vi "UHR-Fleezers Control (fpga) - 10.3.vi"() -> ()   [LabVIEW 2009]
doc: "UHR-Fleezers Instrument Control Code (fpga)"
uses:
  <vilib>/Platform/TimedLoop/XDataNode/XDataNode.xnode
  <vilib>/Platform/TimedLoop/XDataNode/loadlvalarms.vi
  <vilib>/Platform/TimedLoop/XDataNode/timing_clust.ctl
  <vilib>/Platform/TimedLoop/XDataNode/nitl_modes.ctl
  <vilib>/Platform/TimedLoop/XDataNode/wakeup.ctl
  <vilib>/eio/EIONode/EIONode.xnode
  <vilib>/rvi/eio/nirviEIOImplementation/nirviEIOImplementation.xnode
  <vilib>/rvi/eio/common/nirviEmuTemplateMethod_noerrors.vi
  <vilib>/rvi/eio/common/nirviEmuClasses.ctl
  <vilib>/eio/EIOMethodNode/EIOMethodNode.xnode
  <vilib>/rvi/eio/nirviEIOMethodImplementation/nirviEIOMethodImplementation.xnode
  <vilib>/rvi/DataTransferAndStorage/Container/XNode/niFpgaContainer.xnode
  <vilib>/rvi/interface/RandomDataEmulation/niFpgaRandomDataHandleErrors.vi
  <vilib>/rvi/interface/RandomDataEmulation/nirviRandomDataFPGAFIFO.vi
  <vilib>/rvi/DataTransferAndStorage/Container/Common/niFpgaContainerMethod.ctl
  <vilib>/rvi/DataTransferAndStorage/Container/Common/niFpgaTransferTypeControl.ctl
  <vilib>/addons/control/pid/fpga.llb/XNode/niFpgaPID.xnode
  <vilib>/Platform/TimedLoop/XDataNode/XDNodeRunTimeDep.lvlib
panel:
  out "Trap Pos FB Int-Norm Signal":fxp<+/-,16,1> format="%.16g"
  out "Trap Pos FB Int Signal":fxp<+/-,24,9> format="%.18g"
  in  "Tab Control":T1(tab)
  in  "AI1 X Scale":u16
  in  "Trap Pos FB Monitor T1 or T2":bool
  in  "Trap Pos FB Negate Action":bool
  in  "Trap Pos. FB SP":fxp<+/-,16,1>
  in  "Trap Pos. FB Reset":bool
  in  "Trap Pos to FIFO":bool
  in  "AI1 Sets to FIFO":T2={"Set 1"=TRUE, "Set 2"=TRUE, "Set 3"=FALSE}
  in  "N of AI1 Int Acq Sets":i16=2 min=1 max=3 step=1
  out "AI Late Counter":u16
  in  "ai count":u32=400
  out "AI late?":bool
  in  "+ phase":bool
  in  "Phase count adjustment":i16
  out "Relative phase":i16
  in  "AI to FIFO":bool
  out "BD1 Frequency Out 1":u64
  out "BD1 Frequency Out 2":u64
  in  "Force feedback":bool
  out "AI1 X Set 1":fxp<+/-,16,1>
  in  "Trap Pos. FB Gains":T3={"proportional gain (Kc)"=0.0, "integral gain (Kc*Ts/Ti)"=10.0, "derivative gain (Kc*Td/Ts)"=0.0} {"proportional gain (Kc)" format="%.11g"; "integral gain (Kc*Ts/Ti)" format="%.11g"; "derivative gain (Kc*Td/Ts)" format="%.11g"}
  in  "Trap Pos. FB Range":T4={"output high"=0.999969482421875, "output low"=-1.0}
  in  "Trap Pos. FB Mult Factor":i64=2
  in  "Trap Pos. FB Offset Factor":i64
  out "AI1 X Set 2":fxp<+/-,16,1>
  out "Trap Pos FB Action":i64
  out "Trap Pos FIFO Timeout":u16
  out "Trap AI FIFO Timeout":u16
  in  "Trap FIFO Set Timeout":i32
  in  "Trap Pos FB Int Count":u16=100
  in  "Tab Control 2":T5(tab)
  in  "Swap F1 and F2":bool
  in  "Freq or Amp switch first":bool=TRUE
  in  "Cont. Scan":bool
  in  "Abort scan":bool
  in  "Cycles per step":u64
  in  "Scan BD":bool
  in  "Number of scans":u16
  in  "Scan steps":u64
  in  "Scan freq.  increment":i64
  out "Scanning":bool
  in  "Start scan":bool
  in  "OSK Bd 1":bool
  in  "Reset Bd 1":bool
  in  "RD":bool
  in  "PMODE":bool
  in  "OSK Bd 2":bool
  in  "Reset Bd 2":bool
  in  "Direct RF Box \nCommunication":bool
  in  "Data BD 2":u8 format="%08b"
  in  "Data BD 1":u8 format="%08b"
  in  "Address":u8 format="%02x"
  in  "Update Data":bool
  in  "FPGA Controls\n RF Box":bool
  in  "Number Interlace Cycles":u8=2 min=1 max=3
  in  "Interlace Off Parameters":u8=1 min=1 max=3
  in  "Interlace ON/OFF":bool
  out "DIO Relative phase":i16
  in  "Phase count adjustment (DIO)":i16
  in  "+ phase (DIO)":bool
  out "DIO Late Counter":u16
  out "DIO Late?":bool
  in  "DIO count 1 (ticks)":u32=400
  in  "DIO count 2 (ticks)":u32=400
  in  "DIO count 3 (ticks)":u32=400
  out "AI2 Y Sum Set 2":i16
  out "AI2 Y Sum Set 1":i16
  in  "FB Gains Set 1":T6={"proportional gain (Kc)"=10, "integral gain (Kc*Ts/Ti)"=5, "derivative gain (Kc*Td/Ts)"=0}
  in  "FB Setpoint Set 1":i16 min=0 step=1
  in  "FB Reset Set 1":bool
  in  "FB On/Off Set 1":bool
  in  "FB Reset Set 2":bool
  in  "FB On/Off Set 2":bool
  in  "FB Setpoint Set 2":i16 min=0 step=1
  in  "FB Gains Set 2":T6={"proportional gain (Kc)"=10, "integral gain (Kc*Ts/Ti)"=5, "derivative gain (Kc*Td/Ts)"=0}
  in  "FB output range 2":cluster{"output high":i16, "output low":i16}={"output high"=3000, "output low"=0}
  in  "FB output range 1":cluster{"output high":i16, "output low":i16}={"output high"=3000, "output low"=0}
  out "Scan I":u64
  in  "Amp switch delay":u16=5
  in  "Freq switch delay":u16
  in  "BD 2 Amplitude 1":u16
  in  "BD 1 Amplitude 1":u16
  in  "BD 2 Frequency 1":u64
  in  "BD 1 Frequency 1":u64
  in  "BD 2 Amplitude 2":u16
  in  "BD 1 Amplitude 2":u16
  in  "BD 2 Frequency 2":u64
  in  "BD 1 Frequency 2":u64
  in  "BD 2 Amplitude 3":u16
  in  "BD 1 Amplitude 3":u16
  in  "BD 2 Frequency 3":u64
  in  "BD 1 Frequency 3":u64
  out "Numeric":i32
  out "AO2 2":i16
  out "AO1 2":i16
  in  "1D or 2D Scan?":bool
  in  "Abort scan (MCL)":bool
  in  "MCL Scan Axis":bool
  in  "Cont. Scan (MCL)":bool
  out "Scan I (MCL)":u64
  in  "Number of scans (MCL)":u16
  out "Scanning MCL":bool
  in  "Scan steps (MCL)":u64
  in  "Cycles per step (MCL)":u64
  in  "Scan freq.  increment (MCL)":i16
  in  "Start scan (MCL)":bool
  in  "AO2":i16
  in  "AO1":i16
  out "MCL Late Counter":u16
  out "MCL Late?":bool
  in  "MCL count":u32=800
  out "MCL Relative Phase":i16
  in  "Phase count adjustment (MCL)":i16
  in  "+ phase (MCL)":bool
  in  "APD Gate Operating Mode":u8 max=2 step=1
  in  "Invert APD Gate":bool
  in  "APD Gate OFF Count":u32=100
  in  "APD Gate ON Count":u32=300
  out "APD 1 Gate Late Counter":u16
  out "APD 1 Gate Late?":bool
  out "APD 1 Gate Relative Phase":i16
  in  "Phase count adjustment (APD 1 Gate)":i16
  in  "+ phase (APD 1 Gate)":bool
  out "APD 2 Counts 0":u32
  out "APD 2 Counts 1":u32
  out "APD 1 Counts 0":u32
  out "APD 1 Counts 1":u32
  out "APD1 out state":bool
  in  "APD 2 AO scale factor":i16=1
  in  "APD 1 AO scale factor":i16=1
  in  "APD to FIFO":bool
  in  "APD Acq Rate Count":u32=20000000
  out "APD Acq Late Counter":u16
  out "APD Acq Late?":bool
  out "APD Acq Relative Phase":i16
  in  "Phase Count Adjustment (APD Acq)":i16
  in  "+ phase (APD Acq)":bool
  in  "Phase count adjustment (APD 2 Gate)":i16
  out "APD 2 Gate Late Counter":u16
  out "APD 2 Gate Late?":bool
  out "APD 2 Gate Relative Phase":i16
  in  "+ phase (APD 2 Gate)":bool
  out "APD2 out state":bool
  in  "Green Filter Flipper":bool
  out "Green FB Signals":T7
  in  "Green FB Count":u32=1200
  out "Green Late Counter":u16
  out "Green FB Late?":bool
  out "Green FB Relative Phase":i16
  in  "Phase count adjustment (Green FB)":i16=10
  in  "+ phase (Green FB)":bool
  out "Green FB Sum":i16
  in  "Green int current ON count adj":u32=150
  in  "Current Out":u16=30000
  in  "Green FB On/Off":bool
  in  "Green FB Setpoint":i16=250 min=0 step=1
  in  "Green FB Gains":T6={"proportional gain (Kc)"=10, "integral gain (Kc*Ts/Ti)"=5, "derivative gain (Kc*Td/Ts)"=0}
  in  "Green FB Reset":bool
  in  "Operating Mode 2":u8=2 max=2 step=1
  in  "Invert GI 2":bool
  in  "Green interlace OFF count 2":u32=900
  in  "Green interlace ON count 2":u32=300
  out "GI Late Counter 2":u16
  out "GI Late? 2":bool
  out "GI Relative phase 2":i16
  in  "Phase count adjustment (GI) 2":i16=20
  in  "+ phase (GI) 2":bool
  in  "Green interlace OFF count":u32=100
  out "GI Relative phase":i16
  in  "Phase count adjustment (GI)":i16
  in  "+ phase (GI)":bool
  out "GI Late?":bool
  in  "Green interlace ON count":u32=300
  out "GI Late Counter":u16
  in  "Invert GI":bool
  in  "Operating Mode":u8 max=2 step=1
  in  "Chassis2/Mod4/AO1":u16
  # "Only one of these can be on\nat a time:"
  # "Raster Scan AOD"
  # "1 (X)"
  # "2 (Y)"
  # "IR Intensity Feedback (RF BD 1)"
  # "AO1 (Y)"
  # "2D"
  # "1D"
  # "AO2 (X)"
  # "APD AO for aligning"
  # "Detection Loop"
  # "Green fluorescent laser digital gate interlacing loop"
  # "0 Forced ON\n1 Forced OFF\n2 Interlacing"
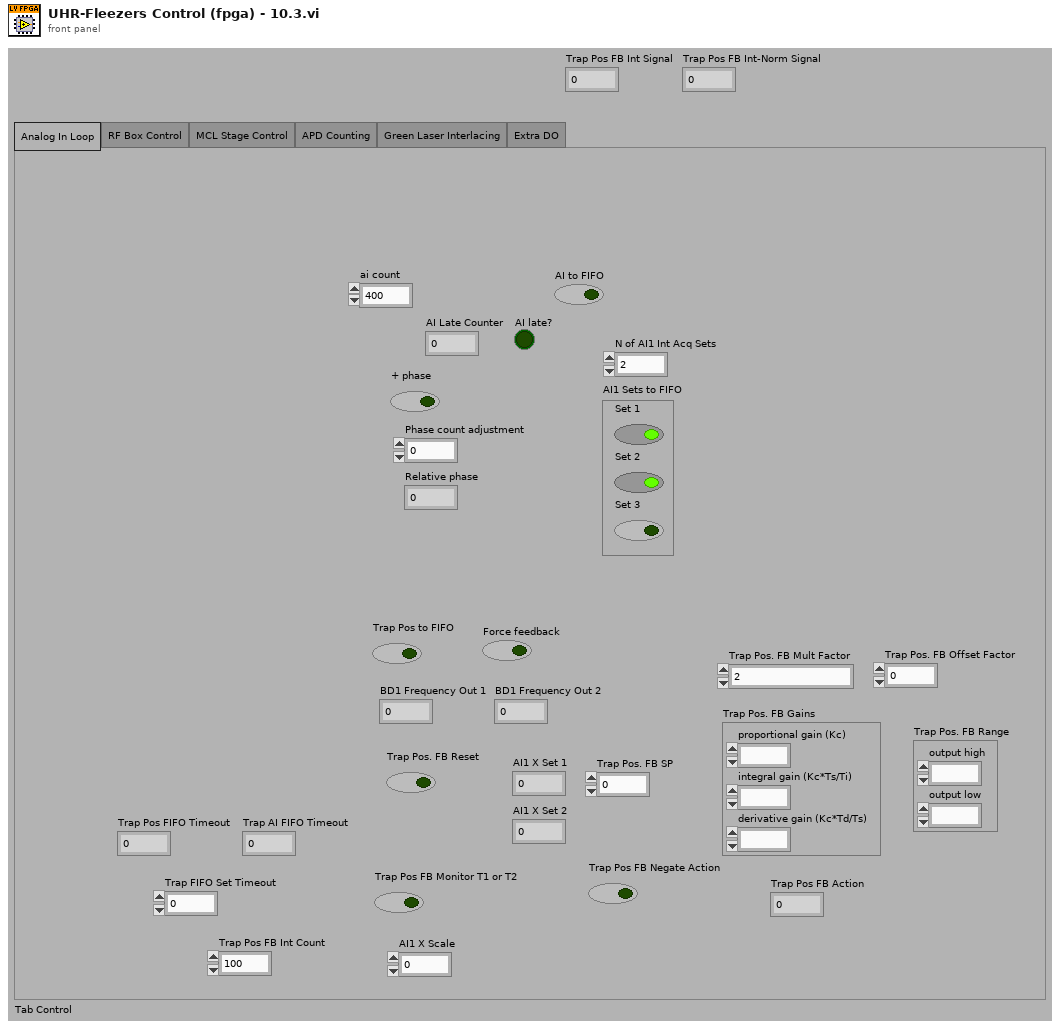
[diagram p1: front panel]
types:
  T1 = enum32{"Analog In Loop", "RF Box Control", "MCL Stage Control", "APD Counting", "Green Laser Interlacing", "Extra DO"}
  T2 = cluster{"Set 1":bool, "Set 2":bool, "Set 3":bool}
  T3 = cluster{"proportional gain (Kc)":fxp<+/-,16,8>, "integral gain (Kc*Ts/Ti)":fxp<+/-,16,8>, "derivative gain (Kc*Td/Ts)":fxp<+/-,16,8>}
  T4 = cluster{"output high":fxp<+/-,16,1>, "output low":fxp<+/-,16,1>}
  T5 = enum32{"Controls", "Interlacing Frequency and Amplitude Values"}
  T6 = cluster{"proportional gain (Kc)":i16, "integral gain (Kc*Ts/Ti)":i16, "derivative gain (Kc*Td/Ts)":i16}
  T7 = cluster{"Green FB Ch 0":i16, "Green FB Ch 1":i16, "Green FB Ch 2":i16}
  T8 = typedef "nirviEmuClasses.ctl" = enum16{"IO Read", "IO Write", "Method", "Property Read", "Property Write"}
  T9 = typedef "XDNodeRunTimeDep.lvlib/timing_clust.ctl" = cluster{"Expected End [f-1]":u64, "Actual End [f-1]":u64, "Finished Late? [f-1]":bool, "Expected End [i-1]":u64, "Actual End [i-1]":u64, "Finished Late? [i-1]":bool, "Expected Start [i]":u64, "Actual Start [i]":u64, "Expected Start [f]":u64, "Actual Start [f]":u64, "Source Name":string, "Structure Name":string, "Period":i64, "Deadline":i64, "Offset":i64, "Start":i64, "Priority":i32, "Timeout":i32, "Mode":T10, "Wakeup Reason":T11, "Error":errorcluster, "Source Type":string, "Secondary Source Type":string, "Global End Time":u64, "Global Start Time":u64, "Frame Duration":u64, "Iteration Duration":u64, "Assigned CPU":i32, "I/O Scan Engine Mode":u32}
  T10 = typedef "XDNodeRunTimeDep.lvlib/nitl_modes.ctl" = enum32{"No Change", "Process missed periods, maintain original phase", "Discard missed periods, maintain original phase", "Process missed periods, ignore original phase", "Discard missed periods, ignore original phase"}
  T11 = typedef "XDNodeRunTimeDep.lvlib/wakeup.ctl" = enum32{"Normal", "Aborted", "Asynchronous wakeup", "Timing source error", "Timed loop error", "Timeout"}
  T12 = typedef "niFpgaContainerMethod.ctl" = enum16{"Write", "Read", "Clear", "Get Number of Elements to Write", "Get Number of Elements to Read", "Enable", "Disable", "Flush and Disable", "Get Stream State"}
  T13 = typedef "niFpgaTransferTypeControl.ctl" = enum16{"Target-Scoped", "Host to Target - DMA", "Target to Host - DMA", "Peer to Peer Reader", "Peer to Peer Writer", "Bidirectional"}
  T14 = cluster{"Chassis2/Mod1/AI0":i16, "Chassis2/Mod1/AI1":i16, "Chassis2/Mod1/AI2":i16}
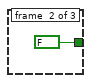
[diagram p2: hidden frame]
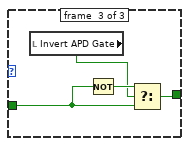
[diagram p3: hidden frame]
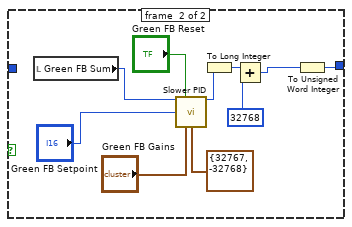
[diagram p4: hidden frame]
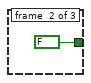
[diagram p5: hidden frame]
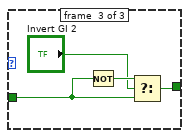
[diagram p6: hidden frame]
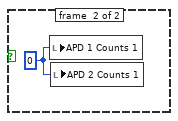
[diagram p7: hidden frame]
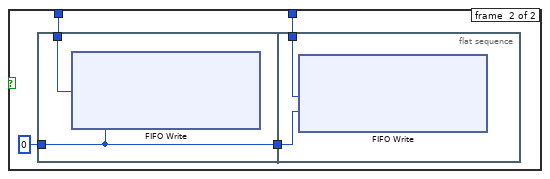
[diagram p8: hidden frame]
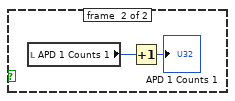
[diagram p9: hidden frame]
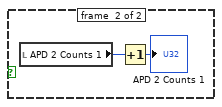
[diagram p10: hidden frame]
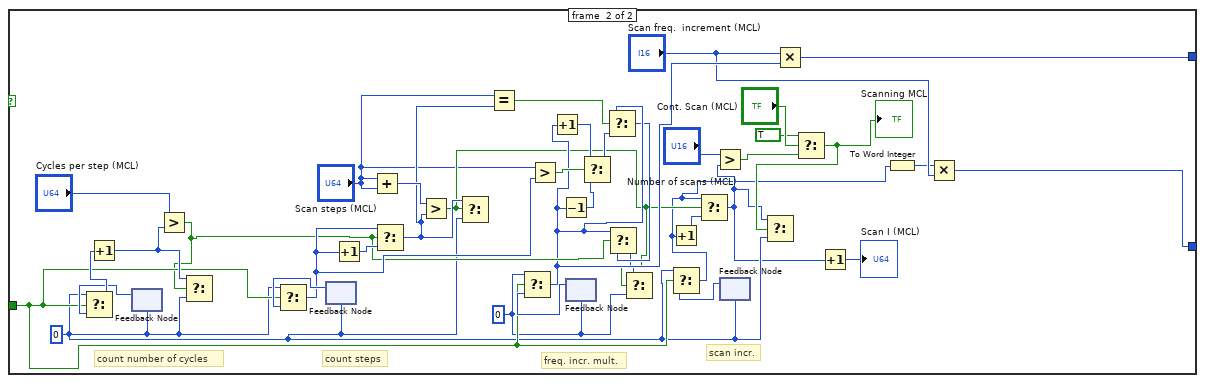
[diagram p11: hidden frame]
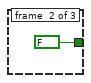
[diagram p12: hidden frame]
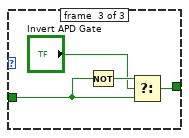
[diagram p13: hidden frame]
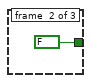
[diagram p14: hidden frame]
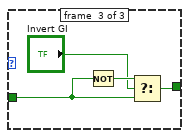
[diagram p15: hidden frame]
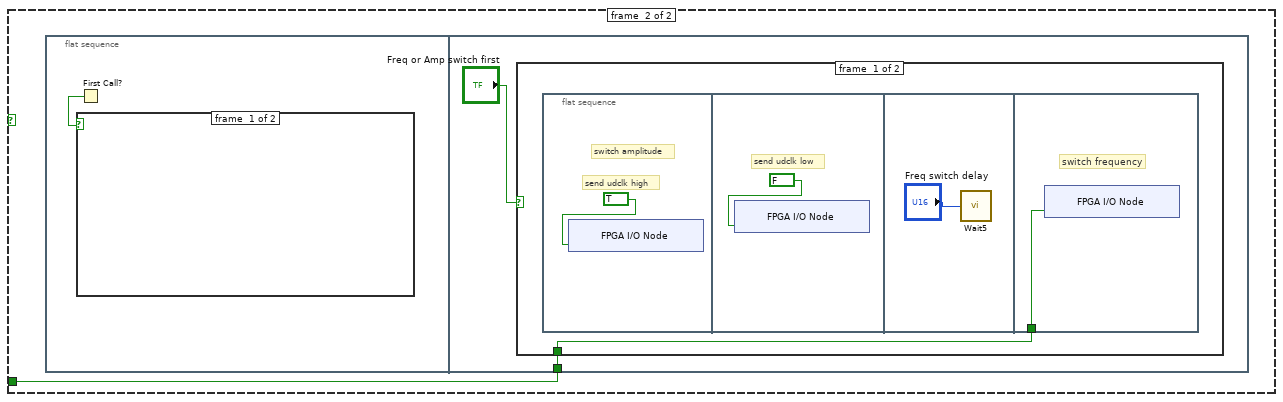
[diagram p16: hidden frame]
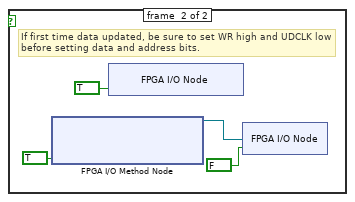
[diagram p17: hidden frame]
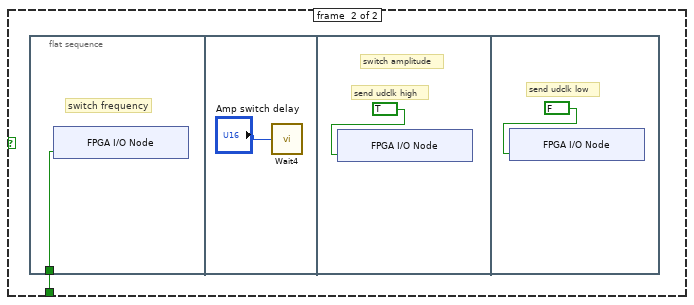
[diagram p18: hidden frame]
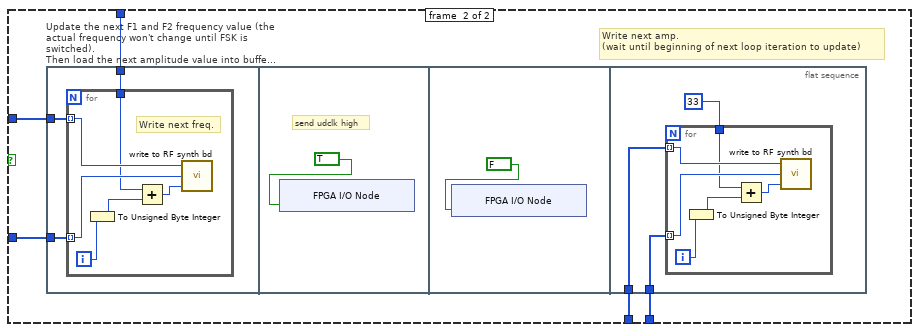
[diagram p19: hidden frame]
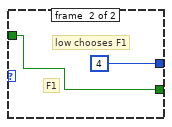
[diagram p20: hidden frame]
diagram:
  w3 = FALSE
  # "timing array current index"
  # "timing array"
  # "timing counter (phase adjusted here)"
  # "late counter"
  n1 = flat-sequence "FPGA initialization to do before running any of the loops" {
    tunnel: [u32 0 ("DIO count 3 (ticks)")] -> w2
    tunnel: [w10] -> _
    frame #0 {
      # "Start up expansion chassis early\nto avoid delays later"
      # "This pin controls udclk on the RF boards.\nWhen initially configuring the boards, this pin needs to be\nconfigured as a high impedance input.  Later it will be switched\nto an output."
      # "Initial setting of DIO data and \naddress to low (before reset).  \nThis needs to happen before the other\ncontrol method loops execute."
      n2 = xnode "FPGA I/O Node"("Chassis2/Mod4/AO0"=u16 0) -> ("Chassis2/Mod1/AI0"=w10:i16)  [unwired: 2 in, 2 out]
      n3 = xnode "FPGA I/O Method Node"("Enable"=FALSE) -> ()  [unwired: 1 in, 1 out]
      n4 = xnode "FPGA I/O Node"("Connector1/DIO0"=FALSE, "Connector1/DIO1"=FALSE, "Connector1/DIO2"=FALSE, "Connector1/DIO3"=FALSE, "Connector1/DIO4"=FALSE, "Connector1/DIO5"=FALSE, "Connector1/DIO6"=FALSE, "Connector1/DIO7"=FALSE, "Connector1/DIO8"=FALSE, "Connector1/DIO9"=FALSE, "Connector1/DIO10"=FALSE, "Connector1/DIO11"=FALSE, "Connector1/DIO12"=FALSE, "Connector1/DIO13"=FALSE, "Connector1/DIO15"=FALSE, "Connector1/DIO20"=FALSE, "Connector1/DIO21"=FALSE, "Connector1/DIO22"=FALSE, "Connector1/DIO23"=FALSE, "Connector1/DIO24"=FALSE, "Connector1/DIO25"=FALSE, "Connector1/DIO26"=FALSE, "Connector1/DIO27"=FALSE, "Connector1/DIO14"=FALSE) -> ()  [unwired: 24 in, 24 out]
    }
  }
  n5 = local read "AO1"() -> (w7:i16)
  n6 = local read "AO2"() -> (w6:i16)
  n7 = node-c288() -> (w5:T9)  [unwired: 1 in]
  n8 = while "APD 1 Counter" {
    tunnel: w2 -> [_]
    stop <- FALSE stop-if-true
    n9 = flat-sequence {
      frame #0 {
        n10 = xnode "FPGA I/O Method Node"("FPGA I/O In"=refnum<k21> "Connector0/DIO0" ("APD 1 DO"), "Timeout"=-1) -> ()  [unwired: 2 out]
      }
      frame #1 {
        n11 = local read "APD1 out state"() -> (w419:bool)
        n12 = case shown="False" w419 {
          frame #0 {
            n13 = local read "APD 1 Counts 0"() -> (w421:u32)
            n14 = Increment(x=w421) -> (x+1=→"APD 1 Counts 0":u32)
          }
          frame #1 {
            n15 = local read "APD 1 Counts 1"() -> (w423:u32)
            n16 = Increment(x=w423) -> (x+1=→"APD 1 Counts 1":u32)
          }
        }
      }
    }
  }
  n17 = while "APD 2 Counter" {
    tunnel: w2 -> [_]
    stop <- FALSE stop-if-true
    n18 = flat-sequence {
      frame #0 {
        n19 = xnode "FPGA I/O Method Node"("FPGA I/O In"=refnum<k21> "Connector0/DIO1" ("APD 2 DO"), "Timeout"=-1) -> ()  [unwired: 2 out]
      }
      frame #1 {
        n20 = local read "APD2 out state"() -> (w450:bool)
        n21 = case shown="False" w450 {
          frame #0 {
            n22 = local read "APD 2 Counts 0"() -> (w452:u32)
            n23 = Increment(x=w452) -> (x+1=→"APD 2 Counts 0":u32)
          }
          frame #1 {
            n24 = local read "APD 2 Counts 1"() -> (w454:u32)
            n25 = Increment(x=w454) -> (x+1=→"APD 2 Counts 1":u32)
          }
        }
      }
    }
  }
  n26 = while "APD 2 Gating" {
    shift-right: [w458] -> _
    shift-left: w2 -> [w463]
    shift-right: [w457] -> _
    shift-left: w3 -> [w455]
    stop <- FALSE stop-if-true
    n27 = flat-sequence {
      tunnel: w463 -> [w466]
      tunnel: [w467] -> w461
      tunnel: [w466] -> w459
      tunnel: [w465] -> w456
      tunnel: w455 -> [w465]
      tunnel: [w470] -> w462
      tunnel: w461 -> [w470]
      tunnel: [w469] -> w460
      tunnel: w459 -> [w469]
      tunnel: w456 -> [w468]
      tunnel: [w532] -> w458
      tunnel: w462 -> [w543]
      tunnel: w460 -> [w541]
      tunnel: [w536] -> w457
      frame #0 {
        n28 = call "Loop Timer8"("Count(Ticks)"=w466) -> ("Tick Count(Ticks)"=w467:u32)
      }
      frame #1 {
        # "(need 4 channels/APD)"
        n29 = xnode "FPGA I/O Node"("Connector0/DIO8"=w468, "Connector0/DIO9"=w468, "Connector0/DIO10"=w468, "Connector0/DIO11"=w468) -> ()  [unwired: 4 in, 4 out]
      }
      frame #2 {
        n30 = local read "APD Gate ON Count"() -> (w525:u32)
        n31 = local read "APD Gate OFF Count"() -> (w524:u32)
        n32 = feedback #1(TRUE) -> (w538:bool)
        n33 = feedback #2(w543) -> (w526:u32)
        n34 = Not(x=w538) -> (.not. x?=w535:bool)
        n35 = Subtract(x=w543, y=w526) -> (x-y=w542:u32)
        n36 = Select(t=w525, s=w535, f=w524) -> (s? t:f=w540:u32)
        n37 = Subtract(x=w542, y=w541) -> (x-y=w517:u32)
        n38 = Subtract(x=w540, y=w517) -> (x-y=w531:u32)
        n39 = Number To Boolean Array(number=w517) -> (Boolean array=w516:bool[])
        n40 = Or Array Elements(Boolean array=w516) -> (logical OR=w515:bool)
        "APD 2 Gate Late?" <- w515
        n41 = Boolean To (0,1)(Boolean="+ phase (APD 2 Gate)") -> (0, 1=w529:i16)
        n42 = Multiply(x=w529, y="Phase count adjustment (APD 2 Gate)") -> (x*y=w527:i16)
        n43 = Boolean To (0,1)(Boolean=w515) -> (0, 1=w522:i16)
        n44 = Add(x=w531, y=w527) -> (x+y=w532:u32)
        n45 = To Unsigned Word Integer(number=w522) -> (unsigned 16bit integer=w519:u16)
        n46 = feedback #3(i16 0) -> (w534:i16)
        n47 = Subtract(x=w534, y=w527) -> (x-y=w533:i16)
        "APD 2 Gate Relative Phase" <- w533
        n48 = feedback #4(u16 0) -> (w520:u16)
        n49 = Add(x=w519, y=w520) -> (x+y=w518:u16)
        "APD 2 Gate Late Counter" <- w518
        n50 = local read "APD Gate Operating Mode"() -> (w523:u8)
        n51 = case shown="2" w523 {
          tunnel: [TRUE FALSE w549] -> w536
          tunnel: w538 -> [_ _ w547]
          frame #0 {
          }
          frame #1 {
          }
          frame #2 {
            n52 = local read "Invert APD Gate"() -> (w546:bool)
            n53 = Not(x=w547) -> (.not. x?=w548:bool)
            n54 = Select(t=w548, s=w546, f=w547) -> (s? t:f=w549:bool)
          }
        }
      }
    }
  }
  n55 = while "DAQ AI set 1" {
    shift-right: [w550] -> _
    shift-left: w2 -> [w555]
    stop <- FALSE stop-if-true
    n56 = flat-sequence {
      tunnel: w555 -> [w565]
      tunnel: [w566] -> w553
      tunnel: [w565] -> w552
      tunnel: [w576] -> w563
      tunnel: [w575] -> w562
      tunnel: [w574] -> w561
      tunnel: [w573] -> w560
      tunnel: [w572] -> w559
      tunnel: [w571] -> w558
      tunnel: [w570] -> w557
      tunnel: [w569] -> w556
      tunnel: [w568] -> w554
      tunnel: w553 -> [w568]
      tunnel: w552 -> [w567]
      tunnel: [w567] -> w551
      tunnel: [w777] -> w550
      tunnel: w563 -> [w805]
      tunnel: w562 -> [w769]
      tunnel: w561 -> [w770]
      tunnel: w560 -> [w804]
      tunnel: w559 -> [w793]
      tunnel: w558 -> [w792]
      tunnel: w557 -> [w791]
      tunnel: w556 -> [w790]
      tunnel: w554 -> [w787]
      tunnel: w551 -> [w784]
      frame #0 {
        n57 = call "Loop Timer3"("Count(Ticks)"=w565) -> ("Tick Count(Ticks)"=w566:u32)
      }
      frame #1 {
        n58 = xnode "FPGA I/O Node"("Connector1/DIO31"=TRUE ("Connector1/DIO33")) -> ("Connector0/AI0"=w576:i16, "Connector0/AI1"=w575:i16, "Connector0/AI2"=w574:i16, "Connector0/AI3"=w573:i16, "Connector0/AI4"=w572:i16, "Connector0/AI5"=w571:i16, "Connector0/AI6"=w570:i16, "Connector0/AI7"=w569:i16)  [unwired: 9 in, 9 out]
      }
      frame #2 {
        w773 = FALSE ("AI to FIFO")
        # "Adjust phase after data acquired if button pressed"
        n59 = feedback #5(i16 1) -> (w797:i16)
        n60 = Increment(x=w797) -> (x+1=w803:i16)
        n61 = Scale By Power Of 2(n="AI1 X Scale", x=w769) -> (x*2^n=w767:i16)
        n62 = Greater?(x=w803, y="N of AI1 Int Acq Sets") -> (0:w800:bool)
        n63 = Divide(x=w767, y=w770) -> (x/y=w766:fxp<+/-,16,1>)
        n64 = Select(t=i16 1, s=w800, f=w803) -> (s? t:f=w802:i16)
        n65 = feedback #6(w773) -> (w771:bool)
        n66 = feedback #7(w773) -> (w789:bool)
        n67 = case shown="1, Default" w797 {
          tunnel: w770 -> [w852 w860 _]
          tunnel: "AI1 Sets to FIFO" -> [w856 w864 w870]
          tunnel: [w855 w863 w869] -> w794
          tunnel: ["AI to FIFO" w862 w868] -> w788
          tunnel: w789 -> [_ w862 w868]
          tunnel: ["Trap Pos to FIFO" w861 w867] -> w772
          tunnel: w771 -> [_ w861 w867]
          tunnel: w766 -> [w851 w859 _]
          tunnel: [w850 w857 FALSE] -> w753
          tunnel: [w849 w858 u64 0 ("BD1 Frequency Out 2")] -> w752
          frame #0 {
            n68 = Unbundle By Name(w856) -> ("Set 1"=w855:bool)
            n69 = local read "BD1 Frequency Out 1"() -> (w849:u64)
            n70 = Compound Arithmetic op=AND("Trap Pos to FIFO", w855, "AI to FIFO") -> (w850:bool)
            "AI2 Y Sum Set 1" <- w852
            "AI1 X Set 1" <- w851
          }
          frame #1 {
            n71 = Unbundle By Name(w864) -> ("Set 2"=w863:bool)
            n72 = local read "BD1 Frequency Out 2"() -> (w858:u64)
            n73 = Compound Arithmetic op=AND(w861, w863, w862) -> (w857:bool)
            "AI2 Y Sum Set 2" <- w860
            "AI1 X Set 2" <- w859
          }
          frame #2 {
            n74 = Unbundle By Name(w870) -> ("Set 3"=w869:bool)
          }
        }
        n75 = And(x=w794, y=w788) -> (x .and. y?=w796:bool)
        n76 = case shown="True" w796 {
          tunnel: w805 -> [_ w884]
          tunnel: w769 -> [_ w883]
          tunnel: w770 -> [_ w882]
          tunnel: w804 -> [_ w881]
          tunnel: w793 -> [_ w880]
          tunnel: w792 -> [_ w879]
          tunnel: w791 -> [_ w878]
          tunnel: w790 -> [_ w877]
          tunnel: 0 ("DMA buffer timeout") -> [_ w886]
          frame #0 {
          }
          frame #1 {
            n77 = Build Array(w884, w883, w882, w881, w880, w879, w878, w877) -> (w885:i16[])
            n78 = for {
              tunnel: w885 -> [w888] mode=indexing
              tunnel: w886 -> [w889]
              tunnel: [w887] -> w875 mode=indexing
              n79 = xnode ("FIFO Write")("Element"=w888, "Timeout"=w889) -> ("Timed Out?"=w887:bool)  [unwired: 1 in, 1 out]
            }
            n80 = Or Array Elements(Boolean array=w875) -> (logical OR=w872:bool)
            n81 = Boolean To (0,1)(Boolean=w872) -> (0, 1=w874:i16)
            n82 = feedback #8(u16 0) -> (w873:u16)
            n83 = Add(x=w874, y=w873) -> (x+y=w871:u16)
            "Trap AI FIFO Timeout" <- w871
          }
        }
        n84 = case shown="True" w753 {
          tunnel: w752 -> [_ w811]
          tunnel: [u8 0 w808] -> w751
          frame #0 {
          }
          frame #1 {
            n85 = Split Number(x=w811) -> (hi(x)=w812:u32, lo(x)=w813:u32)
            n86 = Split Number(x=w812) -> (lo(x)=w814:u16)  [unwired: 1 out]
            n87 = Split Number(x=w813) -> (hi(x)=w815:u16, lo(x)=w816:u16)
            n88 = Build Array "BD 1 nu Stack"(w814, w815, w816) -> (w810:u16[])
            n89 = for {
              tunnel: w810 -> [w823] mode=indexing
              shift-right: [w819] -> w808
              shift-left: u8 0 -> [w820]
              n90 = xnode ("FIFO Method Node")("Element"=w823, "Timeout"="Trap FIFO Set Timeout") -> ("Timed Out?"=w822:bool)  [unwired: 1 in, 1 out]
              n91 = Boolean To (0,1)(Boolean=w822) -> (0, 1=w821:i16)
              n92 = To Unsigned Byte Integer(number=w821) -> (unsigned 8bit integer=w818:u8)
              n93 = Add(x=w818, y=w820) -> (x+y=w819:u8)
            }
          }
        }
        n94 = To Unsigned Word Integer(number=w751) -> (unsigned 16bit integer=w750:u16)
        n95 = feedback #9(u16 0) -> (w764:u16)
        n96 = Add(x=w750, y=w764) -> (x+y=w763:u16)
        "Trap Pos FIFO Timeout" <- w763
        n97 = feedback #10(w787) -> (w786:u32)
        n98 = Subtract(x=w787, y=w786) -> (x-y=w785:u32)
        n99 = xnode "I/O Node"("Connector1/DIO31"=FALSE ("Connector1/DIO34")) -> ()  [unwired: 1 in, 1 out]
        n100 = Subtract(x=w785, y=w784) -> (x-y=w755:u32)
        n101 = Boolean To (0,1)(Boolean="+ phase") -> (0, 1=w780:i16)
        n102 = Multiply(x=w780, y="Phase count adjustment") -> (x*y=w774:i16)
        n103 = Subtract(x="ai count", y=w755) -> (x-y=w778:u32)
        n104 = Number To Boolean Array(number=w755) -> (Boolean array=w756:bool[])
        n105 = feedback #11(i16 0) -> (w776:i16)
        n106 = Add(x=w778, y=w774) -> (x+y=w777:u32)
        n107 = Subtract(x=w776, y=w774) -> (x-y=w775:i16)
        "Relative phase" <- w775
        n108 = Or Array Elements(Boolean array=w756) -> (logical OR=w754:bool)
        "AI late?" <- w754
        n109 = Boolean To (0,1)(Boolean=w754) -> (0, 1=w761:i16)
        n110 = To Unsigned Word Integer(number=w761) -> (unsigned 16bit integer=w758:u16)
        n111 = feedback #12(u16 0) -> (w759:u16)
        n112 = Add(x=w758, y=w759) -> (x+y=w757:u16)
        "AI Late Counter" <- w757
      }
    }
  }
  n113 = while "MCL stage control" {
    shift-right: [w943] -> _
    shift-left: w2 -> [w946]
    shift-right: [w936] -> _
    shift-left: w7 -> [w933]
    shift-right: [w935] -> _
    shift-left: w6 -> [w931]
    i -> [w930]
    stop <- FALSE stop-if-true
    n114 = flat-sequence {
      tunnel: w946 -> [w950]
      tunnel: [w951] -> w942
      tunnel: [w950] -> w940
      tunnel: [w949] -> w934
      tunnel: w933 -> [w949]
      tunnel: [w948] -> w932
      tunnel: w931 -> [w948]
      tunnel: w942 -> [w955]
      tunnel: [w955] -> w941
      tunnel: w940 -> [w954]
      tunnel: [w954] -> w939
      tunnel: w934 -> [w953]
      tunnel: w932 -> [w952]
      tunnel: [w953] -> w929
      tunnel: [w952] -> w928
      tunnel: w941 -> [w989]
      tunnel: w939 -> [w988]
      tunnel: [w989] -> w945
      tunnel: [w988] -> w944
      tunnel: [w987] -> w938
      tunnel: [w986] -> w937
      tunnel: w929 -> [w981]
      tunnel: w928 -> [w980]
      tunnel: [w1061] -> w943
      tunnel: w945 -> [w1068]
      tunnel: w944 -> [w1065]
      tunnel: w938 -> [w1063]
      tunnel: w937 -> [w1062]
      tunnel: [w1063] -> w936
      tunnel: [w1062] -> w935
      frame #0 {
        n115 = call "Loop Timer5"("Count(Ticks)"=w950) -> ("Tick Count(Ticks)"=w951:u32)
      }
      frame #1 {
        n116 = xnode "FPGA I/O Node"("Connector0/AO1"=w953, "Connector0/AO2"=w952) -> ()  [unwired: 2 in, 2 out]
      }
      frame #2 {
        n117 = local read "Scanning MCL"() -> (w1001:bool)
        n118 = Or(x=w1001, y="Start scan (MCL)") -> (x .or. y?=w996:bool)
        n119 = Not(x="Abort scan (MCL)") -> (.not. x?=w994:bool)
        n120 = And(x=w994, y=w996) -> (x .and. y?=w993:bool)
        n121 = case "Raster scan" shown="True" w993 {
          tunnel: [w1002 w1045] -> w998
          tunnel: "Start scan (MCL)" -> [_ w1030]
          tunnel: [w1002 w1006] -> w982
          frame #0 {
            w1002 = i16 0
            n122 = local write "Scanning MCL"(FALSE ("scanning")) -> ()
          }
          frame #1 {
            w1016 = i16 0
            w1015 = u64 0
            # "scan incr."
            # "freq. incr. mult."
            # "count steps"
            # "count number of cycles"
            n123 = feedback #13(w1015) -> (w1042:u64)
            n124 = Select(t=w1015, s=w1030, f=w1042) -> (s? t:f=w1044:u64)
            n125 = Increment(x=w1044) -> (x+1=w1041:u64)
            n126 = Greater?(x="Cycles per step (MCL)", y=w1041) -> (0:w1025:bool)
            n127 = Select(t=w1041, s=w1025, f=w1015) -> (s? t:f=w1040:u64)
            n128 = feedback #14(w1015) -> (w1039:u64)
            n129 = Select(t=w1015, s=w1030, f=w1039) -> (s? t:f=w1034:u64)
            n130 = Increment(x=w1034) -> (x+1=w1038:u64)
            n131 = Add(x="Scan steps (MCL)", y="Scan steps (MCL)") -> (x+y=w1037:u64)
            n132 = Select(t=w1034, s=w1025, f=w1038) -> (s? t:f=w1020:u64)
            n133 = Greater?(x=w1037, y=w1020) -> (0:w1019:bool)
            n134 = Select(t=w1020, s=w1019, f=w1015) -> (s? t:f=w1035:u64)
            n135 = Equal?(x="Scan steps (MCL)", y=w1020) -> (x = y?=w1024:bool)
            n136 = Greater?(x="Scan steps (MCL)", y=w1034) -> (0:w1033:bool)
            n137 = feedback #15(w1016) -> (w1036:i16)
            n138 = Select(t=w1016, s=w1030, f=w1036) -> (s? t:f=w1022:i16)
            n139 = Increment(x=w1022) -> (x+1=w1032:i16)
            n140 = Decrement(x=w1022) -> (x-1=w1031:i16)
            n141 = Select(t=w1032, s=w1033, f=w1031) -> (s? t:f=w1023:i16)
            n142 = Select(t=w1022, s=w1024, f=w1023) -> (s? t:f=w1021:i16)
            n143 = Select(t=w1022, s=w1025, f=w1021) -> (s? t:f=w1017:i16)
            n144 = Select(t=w1017, s=w1019, f=w1016) -> (s? t:f=w1018:i16)
            n145 = feedback #16(w1015) -> (w1029:u64)
            n146 = Select(t=w1015, s=w1030, f=w1029) -> (s? t:f=w1004:u64)
            n147 = Increment(x=w1004) -> (x+1=w1026:u64)
            n148 = Select(t=w1004, s=w1019, f=w1026) -> (s? t:f=w1005:u64)
            n149 = Greater?(x="Number of scans (MCL)", y=w1005) -> (0:w1012:bool)
            n150 = Multiply(x="Scan freq.  increment (MCL)", y=w1022) -> (x*y=w1045:i16)
            n151 = Select(t=TRUE, s="Cont. Scan (MCL)", f=w1012) -> (s? t:f=w1011:bool)
            "Scanning MCL" <- w1011
            n152 = Select(t=w1005, s=w1011, f=w1015) -> (s? t:f=w1027:u64)
            n153 = Increment(x=w1005) -> (x+1=→"Scan I (MCL)":u64)
            n154 = To Word Integer(number=w1004) -> (16bit integer=w1007:i16)
            n155 = Multiply(x=w1007, y="Scan freq.  increment (MCL)") -> (x*y=w1006:i16)
          }
        }
        n156 = Select(t=w982, s="1D or 2D Scan?", f=i16 0) -> (s? t:f=w983:i16)
        n157 = Select(t=w983, s="MCL Scan Axis", f=w998) -> (s? t:f=w997:i16)
        n158 = Select(t=w998, s="MCL Scan Axis", f=w983) -> (s? t:f=w999:i16)
        n159 = Add(x=w997, y="AO2") -> (x+y=w986:i16)
        n160 = Add(x="AO1", y=w999) -> (x+y=w987:i16)
        "AO1 2" <- w981
        "AO2 2" <- w980
      }
      frame #3 {
        n161 = feedback #17(w1068) -> (w1067:u32)
        n162 = Boolean To (0,1)(Boolean="+ phase (MCL)") -> (0, 1=w1059:i16)
        n163 = Subtract(x=w1068, y=w1067) -> (x-y=w1066:u32)
        n164 = Multiply(x=w1059, y="Phase count adjustment (MCL)") -> (x*y=w1055:i16)
        n165 = Subtract(x=w1066, y=w1065) -> (x-y=w1047:u32)
        n166 = Subtract(x="MCL count", y=w1047) -> (x-y=w1057:u32)
        n167 = feedback #18(i16 0) -> (w1056:i16)
        n168 = Subtract(x=w1056, y=w1055) -> (x-y=w1054:i16)
        "MCL Relative Phase" <- w1054
        n169 = Number To Boolean Array(number=w1047) -> (Boolean array=w1048:bool[])
        n170 = Or Array Elements(Boolean array=w1048) -> (logical OR=w1046:bool)
        "MCL Late?" <- w1046
        n171 = Boolean To (0,1)(Boolean=w1046) -> (0, 1=w1053:i16)
        n172 = Add(x=w1057, y=w1055) -> (x+y=w1061:u32)
        n173 = To Unsigned Word Integer(number=w1053) -> (unsigned 16bit integer=w1050:u16)
        n174 = feedback #19(u16 0) -> (w1051:u16)
        n175 = Add(x=w1050, y=w1051) -> (x+y=w1049:u16)
        "MCL Late Counter" <- w1049
      }
    }
    "Numeric" <- w930
  }
  n176 = while "APD 1 Gating" {
    shift-right: [w1073] -> _
    shift-left: w2 -> [w1078]
    shift-right: [w1072] -> _
    shift-left: w3 -> [w1070]
    stop <- FALSE stop-if-true
    n177 = flat-sequence {
      tunnel: w1078 -> [w1081]
      tunnel: [w1082] -> w1076
      tunnel: [w1081] -> w1074
      tunnel: [w1080] -> w1071
      tunnel: w1070 -> [w1080]
      tunnel: [w1085] -> w1077
      tunnel: w1076 -> [w1085]
      tunnel: [w1084] -> w1075
      tunnel: w1074 -> [w1084]
      tunnel: w1071 -> [w1083]
      tunnel: [w1143] -> w1073
      tunnel: w1077 -> [w1158]
      tunnel: w1075 -> [w1155]
      tunnel: [w1147] -> w1072
      frame #0 {
        n178 = call "Loop Timer7"("Count(Ticks)"=w1081) -> ("Tick Count(Ticks)"=w1082:u32)
      }
      frame #1 {
        # "(need 4 channels/APD)"
        n179 = xnode "FPGA I/O Node"("Connector0/DIO4"=w1083, "Connector0/DIO5"=w1083, "Connector0/DIO6"=w1083, "Connector0/DIO7"=w1083) -> ()  [unwired: 4 in, 4 out]
      }
      frame #2 {
        n180 = feedback #20(TRUE) -> (w1150:bool)
        n181 = feedback #21(w1158) -> (w1157:u32)
        n182 = Not(x=w1150) -> (.not. x?=w1146:bool)
        n183 = Subtract(x=w1158, y=w1157) -> (x-y=w1156:u32)
        n184 = Select(t="APD Gate ON Count", s=w1146, f="APD Gate OFF Count") -> (s? t:f=w1152:u32)
        n185 = Subtract(x=w1156, y=w1155) -> (x-y=w1131:u32)
        n186 = Subtract(x=w1152, y=w1131) -> (x-y=w1142:u32)
        n187 = Number To Boolean Array(number=w1131) -> (Boolean array=w1132:bool[])
        n188 = Or Array Elements(Boolean array=w1132) -> (logical OR=w1130:bool)
        "APD 1 Gate Late?" <- w1130
        n189 = Boolean To (0,1)(Boolean="+ phase (APD 1 Gate)") -> (0, 1=w1140:i16)
        n190 = Boolean To (0,1)(Boolean=w1130) -> (0, 1=w1137:i16)
        n191 = Multiply(x=w1140, y="Phase count adjustment (APD 1 Gate)") -> (x*y=w1138:i16)
        n192 = To Unsigned Word Integer(number=w1137) -> (unsigned 16bit integer=w1134:u16)
        n193 = Add(x=w1142, y=w1138) -> (x+y=w1143:u32)
        n194 = feedback #22(i16 0) -> (w1145:i16)
        n195 = Subtract(x=w1145, y=w1138) -> (x-y=w1144:i16)
        "APD 1 Gate Relative Phase" <- w1144
        n196 = feedback #23(u16 0) -> (w1135:u16)
        n197 = Add(x=w1134, y=w1135) -> (x+y=w1133:u16)
        "APD 1 Gate Late Counter" <- w1133
        n198 = case shown="2" "APD Gate Operating Mode" {
          tunnel: [TRUE FALSE w1164] -> w1147
          tunnel: w1150 -> [_ _ w1161]
          frame #0 {
          }
          frame #1 {
          }
          frame #2 {
            n199 = Not(x=w1161) -> (.not. x?=w1163:bool)
            n200 = Select(t=w1163, s="Invert APD Gate", f=w1161) -> (s? t:f=w1164:bool)
          }
        }
      }
    }
  }
  n201 = while "RF box board direct communication loop" {
    tunnel: w2 -> [_]
    stop <- FALSE stop-if-true
    n202 = case "Whether to use direct communication method (only use one method at a time)" shown="True" "Direct RF Box \nCommunication" {
      frame #0 {
      }
      frame #1 {
        n203 = case shown="True" "Update Data" {
          frame #0 {
          }
          frame #1 {
            n204 = flat-sequence {
              frame #0 {
                n205 = First Call?() -> (First Call?: T/F=w1168:bool)
                n206 = case shown="True" w1168 {
                  frame #0 {
                  }
                  frame #1 {
                    # "If first time data updated, be sure to set WR high\nbefore setting data and address bits."
                    n207 = flat-sequence {
                      frame #0 {
                        n208 = xnode "FPGA I/O Node"("Connector1/DIO15"=TRUE) -> ()  [unwired: 1 in, 1 out]
                      }
                      frame #1 {
                        n209 = call "Wait"("Count(Ticks)"=u8 40 ("DO Delay 3 (Ticks)")) -> ()  [unwired: 1 out]
                      }
                    }
                  }
                }
              }
              frame #1 {
                n210 = Number To Boolean Array(number="Address") -> (Boolean array=w1230:bool[])
                n211 = Number To Boolean Array(number="Data BD 1") -> (Boolean array=w1231:bool[])
                n212 = Number To Boolean Array(number="Data BD 2") -> (Boolean array=w1200:bool[])
                n213 = Index Array(array=w1231, index=7) -> (element=w1215:bool)
                n214 = Index Array(array=w1231, index=6) -> (element=w1214:bool)
                n215 = Index Array(array=w1231, index=5) -> (element=w1213:bool)
                n216 = Index Array(array=w1231, index=4) -> (element=w1212:bool)
                n217 = Index Array(array=w1231, index=3) -> (element=w1211:bool)
                n218 = Index Array(array=w1231, index=2) -> (element=w1210:bool)
                n219 = Index Array(array=w1231, index=1) -> (element=w1209:bool)
                n220 = Index Array(array=w1231, index=0) -> (element=w1208:bool)
                n221 = Index Array(array=w1230, index=5) -> (element=w1207:bool)
                n222 = Index Array(array=w1230, index=4) -> (element=w1206:bool)
                n223 = Index Array(array=w1230, index=3) -> (element=w1205:bool)
                n224 = Index Array(array=w1230, index=2) -> (element=w1204:bool)
                n225 = Index Array(array=w1230, index=1) -> (element=w1203:bool)
                n226 = Index Array(array=w1230, index=0) -> (element=w1202:bool)
                n227 = Index Array(array=w1200, index=7) -> (element=w1191:bool)
                n228 = Index Array(array=w1200, index=6) -> (element=w1190:bool)
                n229 = Index Array(array=w1200, index=5) -> (element=w1189:bool)
                n230 = Index Array(array=w1200, index=4) -> (element=w1188:bool)
                n231 = Index Array(array=w1200, index=3) -> (element=w1187:bool)
                n232 = Index Array(array=w1200, index=2) -> (element=w1186:bool)
                n233 = Index Array(array=w1200, index=1) -> (element=w1185:bool)
                n234 = Index Array(array=w1200, index=0) -> (element=w1184:bool)
                n235 = xnode "FPGA I/O Node"("Connector1/DIO0"=w1215, "Connector1/DIO1"=w1214, "Connector1/DIO2"=w1213, "Connector1/DIO3"=w1212, "Connector1/DIO4"=w1211, "Connector1/DIO5"=w1210, "Connector1/DIO6"=w1209, "Connector1/DIO7"=w1208, "Connector1/DIO8"=w1207, "Connector1/DIO9"=w1206, "Connector1/DIO10"=w1205, "Connector1/DIO11"=w1204, "Connector1/DIO12"=w1203, "Connector1/DIO13"=w1202, "Connector1/DIO20"=w1191, "Connector1/DIO21"=w1190, "Connector1/DIO22"=w1189, "Connector1/DIO23"=w1188, "Connector1/DIO24"=w1187, "Connector1/DIO25"=w1186, "Connector1/DIO26"=w1185, "Connector1/DIO27"=w1184) -> ()  [unwired: 22 in, 22 out]
              }
              frame #2 {
                # "wait and then apply write signal"
                n236 = call "Wait2"("Count(Ticks)"=u8 40 ("DO Delay 1 (Ticks)")) -> ()  [unwired: 1 out]
              }
              frame #3 {
                # "sending bit low writes data to board buffer"
                n237 = xnode "FPGA I/O Node"("Connector1/DIO15"=FALSE) -> ()  [unwired: 1 in, 1 out]
              }
              frame #4 {
                # "wait then return write signal"
                n238 = call "Wait3"("Count(Ticks)"=u8 40 ("DO Delay 2 (Ticks)")) -> ()  [unwired: 1 out]
              }
              frame #5 {
                # "sending bit high makes ready to\nwrite more data"
                n239 = xnode "FPGA I/O Node"("Connector1/DIO15"=TRUE) -> ()  [unwired: 1 in, 1 out]
              }
            }
          }
        }
      }
    }
  }
  n240 = while "Control APD data integration - stream to host" {
    shift-right: [w1552] -> _
    shift-left: w2 -> [w1557]
    stop <- FALSE stop-if-true
    n241 = flat-sequence {
      tunnel: w1557 -> [w1559]
      tunnel: [w1560] -> w1555
      tunnel: [w1559] -> w1553
      tunnel: [w1568] -> w1556
      tunnel: w1555 -> [w1568]
      tunnel: [w1567] -> w1554
      tunnel: w1553 -> [w1567]
      tunnel: [w1566] -> w1551
      tunnel: [w1565] -> w1550
      tunnel: [w1602] -> w1552
      tunnel: w1556 -> [w1614]
      tunnel: w1554 -> [w1611]
      tunnel: w1551 -> [w1595]
      tunnel: w1550 -> [w1594]
      frame #0 {
        n242 = call "Loop Timer6"("Count(Ticks)"=w1559) -> ("Tick Count(Ticks)"=w1560:u32)
      }
      frame #1 {
        n243 = flat-sequence {
          tunnel: [w1570] -> w1564
          tunnel: w1564 -> [w1572]
          tunnel: [w1574] -> w1563
          tunnel: [w1573] -> w1562
          tunnel: [w1572] -> w1561
          tunnel: [w1580] -> w1565
          tunnel: [w1581] -> w1566
          tunnel: w1563 -> [w1581]
          tunnel: w1562 -> [w1580]
          tunnel: w1561 -> [w1579]
          frame #0 {
            # "use two separate variable so each APD won't\nhave to wait to read"
            n244 = feedback #24(FALSE) -> (w1569:bool)
            "APD1 out state" <- w1569
            "APD2 out state" <- w1569
            n245 = Not(x=w1569) -> (.not. x?=w1570:bool)
          }
          frame #1 {
            n246 = local read "APD 1 Counts 1"() -> (w1578:u32)
            n247 = local read "APD 1 Counts 0"() -> (w1577:u32)
            n248 = local read "APD 2 Counts 1"() -> (w1576:u32)
            n249 = local read "APD 2 Counts 0"() -> (w1575:u32)
            n250 = Select(t=w1578, s=w1572, f=w1577) -> (s? t:f=w1574:u32)
            n251 = Select(t=w1576, s=w1572, f=w1575) -> (s? t:f=w1573:u32)
          }
          frame #2 {
            n252 = case shown="False" w1579 {
              frame #0 {
                w1582 = u32 0 ("APD 1 Counts 0")
                n253 = local write "APD 1 Counts 0"(w1582) -> ()
                n254 = local write "APD 2 Counts 0"(w1582) -> ()
              }
              frame #1 {
                w1583 = u32 0 ("APD 1 Counts 1")
                n255 = local write "APD 1 Counts 1"(w1583) -> ()
                n256 = local write "APD 2 Counts 1"(w1583) -> ()
              }
            }
          }
        }
      }
      frame #2 {
        n257 = feedback #25(w1614) -> (w1613:u32)
        n258 = Subtract(x=w1614, y=w1613) -> (x-y=w1612:u32)
        n259 = Subtract(x=w1612, y=w1611) -> (x-y=w1587:u32)
        n260 = case shown="True" "APD to FIFO" {
          tunnel: w1595 -> [_ w1641]
          tunnel: w1594 -> [_ w1639]
          frame #0 {
          }
          frame #1 {
            n261 = flat-sequence {
              tunnel: 0 ("Timeout") -> [w1643]
              tunnel: w1641 -> [w1644]
              tunnel: [w1643] -> w1640
              tunnel: w1640 -> [w1671]
              tunnel: w1639 -> [w1670]
              frame #0 {
                n262 = xnode ("FIFO Write")("Element"=w1644, "Timeout"=w1643) -> ()  [unwired: 1 in, 2 out]
              }
              frame #1 {
                n263 = xnode ("FIFO Write")("Element"=w1670, "Timeout"=w1671) -> ()  [unwired: 1 in, 2 out]
              }
            }
          }
        }
        n264 = Subtract(x="APD Acq Rate Count", y=w1587) -> (x-y=w1603:u32)
        n265 = Number To Boolean Array(number=w1587) -> (Boolean array=w1588:bool[])
        n266 = Or Array Elements(Boolean array=w1588) -> (logical OR=w1586:bool)
        "APD Acq Late?" <- w1586
        n267 = Boolean To (0,1)(Boolean=w1586) -> (0, 1=w1593:i16)
        n268 = To Unsigned Word Integer(number=w1593) -> (unsigned 16bit integer=w1590:u16)
        n269 = Boolean To (0,1)(Boolean="+ phase (APD Acq)") -> (0, 1=w1599:i16)
        n270 = feedback #26(u16 0) -> (w1591:u16)
        n271 = Add(x=w1590, y=w1591) -> (x+y=w1589:u16)
        "APD Acq Late Counter" <- w1589
        n272 = Multiply(x=w1599, y="Phase Count Adjustment (APD Acq)") -> (x*y=w1596:i16)
        n273 = Add(x=w1603, y=w1596) -> (x+y=w1602:u32)
        n274 = feedback #27(i16 0) -> (w1601:i16)
        n275 = Subtract(x=w1601, y=w1596) -> (x-y=w1598:i16)
        "APD Acq Relative Phase" <- w1598
        n276 = To Word Integer(number=w1595) -> (16bit integer=w1604:i16)
        n277 = To Word Integer(number=w1594) -> (16bit integer=w1605:i16)
        n278 = Multiply(x="APD 1 AO scale factor", y=w1604) -> (x*y=w1585:i16)
        n279 = Multiply(x="APD 2 AO scale factor", y=w1605) -> (x*y=w1584:i16)
        n280 = xnode "FPGA I/O Node"("Connector0/AO6"=w1585, "Connector0/AO7"=w1584) -> ()  [unwired: 2 in, 2 out]
      }
    }
  }
  n281 = timed-loop "RF box board DIO control: control bits" {
    timing: w5 -> [_]
    timing-out: [_] -> w4
    tunnel: [w1697] -> _
    tunnel: w2 -> [w1697]
    stop <- FALSE stop-if-true
    n282 = xnode "FPGA I/O Node"("Connector1/DIO16"="RD", "Connector1/DIO17"="PMODE", "Connector1/DIO18"="OSK Bd 1", "Connector1/DIO19"="Reset Bd 1", "Connector1/DIO28"="OSK Bd 2", "Connector1/DIO29"="Reset Bd 2") -> ()  [unwired: 6 in, 6 out]
  }
  n283 = while "Green fluorescent laser interlacing (DO to IA 532 nm AOM ME amp)." {
    shift-right: [w1788] -> _
    shift-left: w2 -> [w1793]
    shift-right: [w1787] -> _
    shift-left: FALSE -> [w1785]
    stop <- FALSE stop-if-true
    n284 = flat-sequence {
      tunnel: w1793 -> [w1796]
      tunnel: [w1797] -> w1791
      tunnel: [w1796] -> w1789
      tunnel: [w1795] -> w1786
      tunnel: w1785 -> [w1795]
      tunnel: [w1800] -> w1792
      tunnel: w1791 -> [w1800]
      tunnel: [w1799] -> w1790
      tunnel: w1789 -> [w1799]
      tunnel: w1786 -> [w1798]
      tunnel: [w1848] -> w1788
      tunnel: w1792 -> [w1868]
      tunnel: w1790 -> [w1865]
      tunnel: [w1857] -> w1787
      frame #0 {
        n285 = call "Loop Timer4"("Count(Ticks)"=w1796) -> ("Tick Count(Ticks)"=w1797:u32)
      }
      frame #1 {
        n286 = xnode "FPGA I/O Node"("Connector1/DIO37"=w1798, "Connector1/DIO38"=w1798, "Connector1/DIO39"=w1798) -> ()  [unwired: 3 in, 3 out]
      }
      frame #2 {
        n287 = feedback #28(w1868) -> (w1867:u32)
        n288 = Subtract(x=w1868, y=w1867) -> (x-y=w1866:u32)
        n289 = Subtract(x=w1866, y=w1865) -> (x-y=w1841:u32)
        n290 = Number To Boolean Array(number=w1841) -> (Boolean array=w1842:bool[])
        n291 = Or Array Elements(Boolean array=w1842) -> (logical OR=w1840:bool)
        "GI Late?" <- w1840
        n292 = Boolean To (0,1)(Boolean="+ phase (GI)") -> (0, 1=w1853:i16)
        n293 = Multiply(x=w1853, y="Phase count adjustment (GI)") -> (x*y=w1850:i16)
        n294 = Boolean To (0,1)(Boolean=w1840) -> (0, 1=w1847:i16)
        n295 = To Unsigned Word Integer(number=w1847) -> (unsigned 16bit integer=w1844:u16)
        n296 = feedback #29(i16 0) -> (w1851:i16)
        n297 = feedback #30(u16 0) -> (w1845:u16)
        n298 = Add(x=w1844, y=w1845) -> (x+y=w1843:u16)
        "GI Late Counter" <- w1843
        n299 = Subtract(x=w1851, y=w1850) -> (x-y=w1849:i16)
        "GI Relative phase" <- w1849
        n300 = feedback #31(TRUE) -> (w1860:bool)
        n301 = case shown="2" "Operating Mode" {
          tunnel: [TRUE FALSE w1874] -> w1857
          tunnel: w1860 -> [_ _ w1871]
          frame #0 {
          }
          frame #1 {
          }
          frame #2 {
            n302 = Not(x=w1871) -> (.not. x?=w1873:bool)
            n303 = Select(t=w1873, s="Invert GI", f=w1871) -> (s? t:f=w1874:bool)
          }
        }
        n304 = Not(x=w1860) -> (.not. x?=w1856:bool)
        n305 = Select(t="Green interlace ON count", s=w1856, f="Green interlace OFF count") -> (s? t:f=w1862:u32)
        n306 = Subtract(x=w1862, y=w1841) -> (x-y=w1854:u32)
        n307 = Add(x=w1854, y=w1850) -> (x+y=w1848:u32)
      }
    }
  }
  n308 = while "Green fluorescent laser interlacing (Current to IA 532 nm AOM ME amp)." {
    shift-right: [w1880] -> _
    shift-left: w2 -> [w1883]
    shift-right: [w1877] -> _
    shift-left: u16 0 -> [w1875]
    stop <- FALSE stop-if-true
    n309 = flat-sequence {
      tunnel: w1883 -> [w1886]
      tunnel: [w1887] -> w1882
      tunnel: [w1886] -> w1881
      tunnel: [w1885] -> w1876
      tunnel: w1875 -> [w1885]
      tunnel: [w1890] -> w1879
      tunnel: w1882 -> [w1890]
      tunnel: [w1889] -> w1878
      tunnel: w1881 -> [w1889]
      tunnel: w1876 -> [w1888]
      tunnel: [w1911] -> w1880
      tunnel: [w1928] -> w1877
      tunnel: w1879 -> [w1941]
      tunnel: w1878 -> [w1938]
      frame #0 {
        n310 = call "Loop Timer10"("Count(Ticks)"=w1886) -> ("Tick Count(Ticks)"=w1887:u32)
      }
      frame #1 {
        n311 = xnode "FPGA I/O Node"("Chassis2/Mod4/AO0"=w1888) -> ()  [unwired: 1 in, 1 out]
      }
      frame #2 {
        n312 = Subtract(x="Green interlace OFF count 2", y="Green int current ON count adj") -> (x-y=w1920:u32)
        n313 = feedback #32(w1941) -> (w1940:u32)
        n314 = Add(x="Green int current ON count adj", y="Green interlace ON count 2") -> (x+y=w1921:u32)
        n315 = Subtract(x=w1941, y=w1940) -> (x-y=w1939:u32)
        n316 = Subtract(x=w1939, y=w1938) -> (x-y=w1904:u32)
        n317 = Number To Boolean Array(number=w1904) -> (Boolean array=w1905:bool[])
        n318 = Boolean To (0,1)(Boolean="+ phase (GI) 2") -> (0, 1=w1917:i16)
        n319 = Or Array Elements(Boolean array=w1905) -> (logical OR=w1903:bool)
        "GI Late? 2" <- w1903
        n320 = Boolean To (0,1)(Boolean=w1903) -> (0, 1=w1910:i16)
        n321 = Multiply(x=w1917, y="Phase count adjustment (GI) 2") -> (x*y=w1913:i16)
        n322 = To Unsigned Word Integer(number=w1910) -> (unsigned 16bit integer=w1906:u16)
        n323 = feedback #33(u16 0) -> (w1908:u16)
        n324 = Add(x=w1906, y=w1908) -> (x+y=w1907:u16)
        "GI Late Counter 2" <- w1907
        n325 = feedback #34(i16 0) -> (w1914:i16)
        n326 = Subtract(x=w1914, y=w1913) -> (x-y=w1912:i16)
        "GI Relative phase 2" <- w1912
        n327 = feedback #35(TRUE) -> (w1933:bool)
        n328 = case shown="2" "Operating Mode 2" {
          tunnel: [TRUE FALSE w1958] -> w1922
          tunnel: w1933 -> [_ _ w1955]
          frame #0 {
          }
          frame #1 {
          }
          frame #2 {
            n329 = Not(x=w1955) -> (.not. x?=w1957:bool)
            n330 = Select(t=w1957, s="Invert GI 2", f=w1955) -> (s? t:f=w1958:bool)
          }
        }
        n331 = And(x=w1922, y="Green FB On/Off") -> (x .and. y?=w1923:bool)
        n332 = case shown="True" w1923 {
          tunnel: "Current Out" -> [w1942 _]
          tunnel: [w1942 w1947] -> w1927
          frame #0 {
          }
          frame #1 {
            n333 = local read "Green FB Sum"() -> (w1943:i16)
            n334 = call "Slower PID.vi"("process variable"=w1943, "reset?"="Green FB Reset", "setpoint"="Green FB Setpoint", "PID gains (x 2^8)"="Green FB Gains", "output range"=cluster{"output high":i16, "output low":i16} {"output high"=32767, "output low"=-32768} ("Green FB output range")) -> ("output"=w1951:i16)  [unwired: 10 out]
            n335 = To Long Integer(number=w1951) -> (32bit integer=w1944:i32)
            n336 = Add(x=w1944, y=32768) -> (x+y=w1946:i32)
            n337 = To Unsigned Word Integer(number=w1946) -> (unsigned 16bit integer=w1947:u16)
          }
        }
        n338 = Not(x=w1933) -> (.not. x?=w1930:bool)
        n339 = Select(t=w1921, s=w1930, f=w1920) -> (s? t:f=w1935:u32)
        n340 = Subtract(x=w1935, y=w1904) -> (x-y=w1915:u32)
        n341 = Add(x=w1915, y=w1913) -> (x+y=w1911:u32)
        n342 = Boolean To (0,1)(Boolean=w1922) -> (0, 1=w1929:i16)
        n343 = To Unsigned Word Integer(number=w1929) -> (unsigned 16bit integer=w1926:u16)
        n344 = Multiply(x=w1926, y=w1927) -> (x*y=w1928:u16)
      }
    }
  }
  n345 = while "Green excitation laser feedback measurement" {
    shift-right: [w1959] -> _
    shift-left: w2 -> [w1964]
    stop <- FALSE stop-if-true
    n346 = flat-sequence {
      tunnel: w1964 -> [w1966]
      tunnel: [w1967] -> w1962
      tunnel: [w1966] -> w1960
      tunnel: [w1974] -> w1963
      tunnel: w1962 -> [w1974]
      tunnel: [w1973] -> w1961
      tunnel: w1960 -> [w1973]
      tunnel: [w2058] -> w1959
      tunnel: w1963 -> [w2069]
      tunnel: w1961 -> [w2066]
      frame #0 {
        n347 = call "Loop Timer9"("Count(Ticks)"=w1966) -> ("Tick Count(Ticks)"=w1967:u32)
      }
      frame #1 {
        n348 = xnode "FPGA I/O Node"("Connector1/DIO35"=TRUE) -> ("Chassis2/Mod1/AI0"=w1972:i16, "Chassis2/Mod1/AI1"=w1971:i16, "Chassis2/Mod1/AI2"=w1968:i16)  [unwired: 4 in, 4 out]
        "Green FB Sum" <- w1968
        n349 = Bundle("Chassis2/Mod1/AI0"=w1972, "Chassis2/Mod1/AI1"=w1971, "Chassis2/Mod1/AI2"=w1968) -> (→"Green FB Signals":T14)  [unwired: 1 out]
      }
      frame #2 {
        n350 = feedback #36(w2069) -> (w2068:u32)
        n351 = Subtract(x=w2069, y=w2068) -> (x-y=w2067:u32)
        n352 = xnode "FPGA I/O Node"("Connector1/DIO35"=FALSE) -> ()  [unwired: 1 in, 1 out]
        n353 = Subtract(x=w2067, y=w2066) -> (x-y=w2048:u32)
        n354 = Subtract(x="Green FB Count", y=w2048) -> (x-y=w2062:u32)
        n355 = Number To Boolean Array(number=w2048) -> (Boolean array=w2049:bool[])
        n356 = Or Array Elements(Boolean array=w2049) -> (logical OR=w2047:bool)
        "Green FB Late?" <- w2047
        n357 = Boolean To (0,1)(Boolean="+ phase (Green FB)") -> (0, 1=w2060:i16)
        n358 = Boolean To (0,1)(Boolean=w2047) -> (0, 1=w2054:i16)
        n359 = Multiply(x=w2060, y="Phase count adjustment (Green FB)") -> (x*y=w2055:i16)
        n360 = Add(x=w2062, y=w2055) -> (x+y=w2058:u32)
        n361 = To Unsigned Word Integer(number=w2054) -> (unsigned 16bit integer=w2051:u16)
        n362 = feedback #37(i16 0) -> (w2057:i16)
        n363 = Subtract(x=w2057, y=w2055) -> (x-y=w2056:i16)
        "Green FB Relative Phase" <- w2056
        n364 = feedback #38(u16 0) -> (w2052:u16)
        n365 = Add(x=w2051, y=w2052) -> (x+y=w2050:u16)
        "Green Late Counter" <- w2050
      }
    }
  }
  n366 = while "Control Additional IO (Green laser flip mount)" {
    stop <- FALSE stop-if-true
    n367 = xnode "FPGA I/O Node"("Connector0/DIO3"="Green Filter Flipper", "Chassis2/Mod4/AO1"="Chassis2/Mod4/AO1") -> ()  [unwired: 2 in, 2 out]
    n368 = call "Loop Timer2"("Count(Ticks)"=u32 40000 ("Extra DO Counts")) -> ()  [unwired: 1 out]
  }
  n369 = while "RF box board DIO control: parallel communication" {
    shift-right: [w2114] -> _
    shift-left: w2 -> [w2113]
    shift-right: [w2112] -> _
    shift-left: FALSE ("Swap F1 and F2") -> [w2111]
    stop <- FALSE stop-if-true
    n370 = flat-sequence {
      tunnel: w2111 -> [w2118]
      tunnel: w2113 -> [w2116]
      tunnel: [w2118] -> w2110
      tunnel: [w2117] -> w2109
      tunnel: [w2116] -> w2108
      tunnel: [w2124] -> w2114
      tunnel: [w2123] -> w2112
      tunnel: w2110 -> [w2122]
      tunnel: w2109 -> [w2120]
      tunnel: w2108 -> [w2119]
      frame #0 {
        n371 = call "Loop Timer"("Count(Ticks)"=w2116) -> ("Tick Count(Ticks)"=w2117:u32)
      }
      frame #1 {
        n372 = flat-sequence {
          tunnel: ["FPGA Controls\n RF Box"] -> w2121
          tunnel: w2122 -> [w2125]
          tunnel: [w2282] -> w2124
          tunnel: [w2295] -> w2123
          tunnel: w2121 -> [w2294]
          tunnel: w2120 -> [w2288]
          tunnel: w2119 -> [w2285]
          frame #0 {
            n373 = case shown="True" "FPGA Controls\n RF Box" {
              tunnel: w2125 -> [_ w2127]
              frame #0 {
              }
              frame #1 {
                n374 = flat-sequence {
                  tunnel: w2127 -> [w2172]
                  frame #0 {
                    n375 = First Call?() -> (First Call?: T/F=w2128:bool)
                    n376 = case shown="True" w2128 {
                      frame #0 {
                      }
                      frame #1 {
                        # "If first time data updated, be sure to set WR high and UDCLK low\nbefore setting data and address bits."
                        n377 = xnode "FPGA I/O Method Node"("Enable"=TRUE) -> ("FPGA I/O Out"=w2130:refnum<k21>)  [unwired: 1 in]
                        n378 = xnode "FPGA I/O Node"("Connector1/DIO15"=TRUE) -> ()  [unwired: 1 in, 1 out]
                        n379 = xnode "FPGA I/O Node"("I/O Item"=FALSE ("Connector1/DIO30"), "FPGA I/O In"=w2130) -> ()  [unwired: 1 out]
                      }
                    }
                  }
                  frame #1 {
                    n380 = case shown="True" "Freq or Amp switch first" {
                      tunnel: w2172 -> [w2174 w2218]
                      frame #0 {
                        n381 = flat-sequence {
                          tunnel: w2174 -> [w2204]
                          frame #0 {
                            # "switch amplitude"
                            # "send udclk high"
                            n382 = xnode "FPGA I/O Node"("Connector1/DIO30"=TRUE ("Connector1/DIO15")) -> ()  [unwired: 1 in, 1 out]
                          }
                          frame #1 {
                            # "send udclk low"
                            n383 = xnode "FPGA I/O Node"("Connector1/DIO30"=FALSE ("Connector1/DIO15")) -> ()  [unwired: 1 in, 1 out]
                          }
                          frame #2 {
                            n384 = call "Wait5"("Count(Ticks)"="Freq switch delay") -> ()  [unwired: 1 out]
                          }
                          frame #3 {
                            # "switch frequency"
                            n385 = xnode "FPGA I/O Node"("Connector1/DIO36"=w2204) -> ()  [unwired: 1 in, 1 out]
                          }
                        }
                      }
                      frame #1 {
                        n386 = flat-sequence {
                          tunnel: w2218 -> [w2219]
                          frame #0 {
                            # "switch frequency"
                            n387 = xnode "FPGA I/O Node"("Connector1/DIO36"=w2219) -> ()  [unwired: 1 in, 1 out]
                          }
                          frame #1 {
                            n388 = call "Wait4"("Count(Ticks)"="Amp switch delay") -> ()  [unwired: 1 out]
                          }
                          frame #2 {
                            # "switch amplitude"
                            # "send udclk high"
                            n389 = xnode "FPGA I/O Node"("Connector1/DIO30"=TRUE ("Connector1/DIO15")) -> ()  [unwired: 1 in, 1 out]
                          }
                          frame #3 {
                            # "send udclk low"
                            n390 = xnode "FPGA I/O Node"("Connector1/DIO30"=FALSE ("Connector1/DIO15")) -> ()  [unwired: 1 in, 1 out]
                          }
                        }
                      }
                    }
                  }
                }
              }
            }
          }
          frame #1 {
            # "This is the prior cycle's on time"
            # "increment timing\nindex, reset to 0 if \nend of matrix"
            # "Reset to begginning (1) when number of cycles reached."
            # "timing index"
            # "build byte stacks for writing data\n(must correspond to addresses array constant)"
            # "Timing housekeeping"
            # "Adjust phase if late\n(maintains constant phase relationship between cycles)"
            n391 = feedback #39(u8 0 ("t")) -> (w2291:u8)
            n392 = Increment(x=w2291) -> (x+1=w2335:u8)
            n393 = Increment(x="Number Interlace Cycles") -> (x+1=w2330:u8)
            n394 = Equal?(x=w2335, y=w2330) -> (x = y?=w2337:bool)
            n395 = Select(t=u8 1, s=w2337, f=w2335) -> (s? t:f=w2290:u8)
            n396 = Increment(x=w2290) -> (x+1=w2332:u8)
            n397 = Equal?(x=w2332, y=w2330) -> (x = y?=w2333:bool)
            n398 = Select(t=u8 1, s=w2333, f=w2332) -> (s? t:f=w2329:u8)
            n399 = Select(t=w2329, s="Interlace ON/OFF", f="Interlace Off Parameters") -> (s? t:f=w2313:u8)
            n400 = case shown="1, Default" w2313 {
              tunnel: [w2412 "BD 1 Frequency 2" "BD 1 Frequency 3"] -> w2325
              tunnel: [w2411 "BD 2 Frequency 2" "BD 2 Frequency 3"] -> w2314
              tunnel: ["BD 2 Amplitude 1" "BD 2 Amplitude 2" "BD 2 Amplitude 3"] -> w2270
              tunnel: [w2400 w2545 "BD 1 Amplitude 3"] -> w2273
              frame #0 {
                w2407 = u64 0 ("f")
                # "Trap 1"
                n401 = local read "Scanning"() -> (w2413:bool)
                n402 = case "For position feedback" shown="True" "Force feedback" {
                  tunnel: [i64 0 w2431] -> w2397
                  frame #0 {
                  }
                  frame #1 {
                    w2422 = fxp<+/-,24,9> 0.0 ("AI1 X Set 2")
                    w2434 = u16 0
                    n403 = local read "AI1 X Set 2"() -> (w2428:fxp<+/-,16,1>)
                    n404 = local read "AI1 X Set 1"() -> (w2427:fxp<+/-,16,1>)
                    n405 = feedback #40(w2434) -> (w2435:u16)
                    n406 = Increment(x=w2435) -> (x+1=w2433:u16)
                    n407 = Select(t=w2427, s="Trap Pos FB Monitor T1 or T2", f=w2428) -> (s? t:f=w2424:fxp<+/-,16,1>)
                    n408 = Greater Or Equal?(x=w2433, y="Trap Pos FB Int Count") -> (x >= y?=w2425:bool)
                    n409 = Select(t=w2434, s=w2425, f=w2433) -> (s? t:f=w2432:u16)
                    n410 = feedback #41(w2422) -> (w2423:fxp<+/-,24,9>)
                    n411 = Add(x=w2424, y=w2423) -> (x+y=w2419:fxp<+/-,24,9>)
                    n412 = Select(t=w2422, s=w2425, f=w2419) -> (s? t:f=w2421:fxp<+/-,24,9>)
                    n413 = feedback #42(i64 0) -> (w2430:i64)
                    n414 = case shown="True" w2425 {
                      tunnel: [w2436 w2450] -> w2431
                      tunnel: w2430 -> [w2436 _]
                      tunnel: "Trap Pos FB Int Count" -> [_ w2438]
                      tunnel: w2419 -> [_ w2439]
                      frame #0 {
                      }
                      frame #1 {
                        n415 = Divide(x=w2439, y=w2438) -> (x/y=w2437:fxp<+/-,16,1>)
                        "Trap Pos FB Int-Norm Signal" <- w2437
                        n416 = xnode ("PID")("process variable"=w2437, "reset?"="Trap Pos. FB Reset", "setpoint"="Trap Pos. FB SP", "PID gains"="Trap Pos. FB Gains", "output range"="Trap Pos. FB Range") -> ("output"=w2448:fxp<+/-,16,1>)
                        n417 = Negate(x=w2448) -> (-x=w2447:fxp<+/-,17,2>)
                        n418 = Select(t=w2447, s="Trap Pos FB Negate Action", f=w2448) -> (s? t:f=w2444:fxp<+/-,17,2>)
                        n419 = Scale By Power Of 2(n=u32 15, x=u32 1) -> (x*2^n=w2441:u32)
                        n420 = Multiply(x=w2444, y=w2441) -> (x*y=w2440:fxp<+/-,17,17>)
                        n421 = To Quad Integer(1:w2440) -> (0:w2453:i64)
                        "Trap Pos FB Action" <- w2453
                        n422 = Multiply(x=w2453, y="Trap Pos. FB Mult Factor") -> (x*y=w2451:i64)
                        n423 = Add(x=w2451, y="Trap Pos. FB Offset Factor") -> (x+y=w2450:i64)
                        "Trap Pos FB Int Signal" <- w2439
                      }
                    }
                  }
                }
                n424 = Or(x=w2413, y="Start scan") -> (x .or. y?=w2405:bool)
                n425 = Not(x="Abort scan") -> (.not. x?=w2403:bool)
                n426 = And(x=w2403, y=w2405) -> (x .and. y?=w2402:bool)
                n427 = case "For raster scanning" shown="False" w2402 {
                  tunnel: [u64 0 w2533] -> w2408
                  tunnel: "Start scan" -> [_ w2518]
                  frame #0 {
                    n428 = local write "Scanning"(FALSE ("scanning")) -> ()
                  }
                  frame #1 {
                    w2502 = i64 0
                    w2501 = u64 0
                    # "scan incr."
                    # "freq. incr. mult."
                    # "count steps"
                    # "count number of cycles"
                    n429 = feedback #43(w2501) -> (w2530:u64)
                    n430 = Select(t=w2501, s=w2518, f=w2530) -> (s? t:f=w2532:u64)
                    n431 = Increment(x=w2532) -> (x+1=w2529:u64)
                    n432 = Greater?(x="Cycles per step", y=w2529) -> (0:w2511:bool)
                    n433 = Select(t=w2529, s=w2511, f=w2501) -> (s? t:f=w2528:u64)
                    n434 = feedback #44(w2501) -> (w2527:u64)
                    n435 = Select(t=w2501, s=w2518, f=w2527) -> (s? t:f=w2522:u64)
                    n436 = Increment(x=w2522) -> (x+1=w2526:u64)
                    n437 = Add(x="Scan steps", y="Scan steps") -> (x+y=w2525:u64)
                    n438 = Select(t=w2522, s=w2511, f=w2526) -> (s? t:f=w2506:u64)
                    n439 = Greater?(x=w2525, y=w2506) -> (0:w2505:bool)
                    n440 = Select(t=w2506, s=w2505, f=w2501) -> (s? t:f=w2523:u64)
                    n441 = Equal?(x="Scan steps", y=w2506) -> (x = y?=w2510:bool)
                    n442 = Greater?(x="Scan steps", y=w2522) -> (0:w2521:bool)
                    n443 = feedback #45(w2502) -> (w2524:i64)
                    n444 = Select(t=w2502, s=w2518, f=w2524) -> (s? t:f=w2508:i64)
                    n445 = Increment(x=w2508) -> (x+1=w2520:i64)
                    n446 = Decrement(x=w2508) -> (x-1=w2519:i64)
                    n447 = Select(t=w2520, s=w2521, f=w2519) -> (s? t:f=w2509:i64)
                    n448 = Select(t=w2508, s=w2510, f=w2509) -> (s? t:f=w2507:i64)
                    n449 = Select(t=w2508, s=w2511, f=w2507) -> (s? t:f=w2503:i64)
                    n450 = Select(t=w2503, s=w2505, f=w2502) -> (s? t:f=w2504:i64)
                    n451 = feedback #46(w2501) -> (w2517:u64)
                    n452 = Select(t=w2501, s=w2518, f=w2517) -> (s? t:f=w2513:u64)
                    n453 = Increment(x=w2513) -> (x+1=w2514:u64)
                    n454 = Select(t=w2513, s=w2505, f=w2514) -> (s? t:f=w2512:u64)
                    n455 = Greater?(x="Number of scans", y=w2512) -> (0:w2498:bool)
                    n456 = Multiply(x="Scan freq.  increment", y=w2508) -> (x*y=w2533:i64)
                    n457 = Select(t=TRUE, s="Cont. Scan", f=w2498) -> (s? t:f=w2497:bool)
                    "Scanning" <- w2497
                    n458 = Select(t=w2512, s=w2497, f=w2501) -> (s? t:f=w2515:u64)
                    n459 = Increment(x=w2512) -> (x+1=→"Scan I":u64)
                  }
                }
                n460 = case "For intensity feedback" shown="True" "FB On/Off Set 1" {
                  tunnel: "BD 1 Amplitude 1" -> [w2535 _]
                  tunnel: [w2535 w2536] -> w2400
                  frame #0 {
                  }
                  frame #1 {
                    n461 = local read "AI2 Y Sum Set 1"() -> (w2538:i16)
                    n462 = call "Slower PID.vi"("process variable"=w2538, "reset?"="FB Reset Set 1", "setpoint"="FB Setpoint Set 1", "PID gains (x 2^8)"="FB Gains Set 1", "output range"="FB output range 1") -> ("output"=w2541:i16)  [unwired: 10 out]
                    n463 = To Unsigned Word Integer(number=w2541) -> (unsigned 16bit integer=w2536:u16)
                  }
                }
                n464 = Select(t=w2407, s="Scan BD", f=w2408) -> (s? t:f=w2406:u64)
                n465 = Select(t=w2408, s="Scan BD", f=w2407) -> (s? t:f=w2409:u64)
                n466 = Add(x=w2406, y="BD 2 Frequency 1") -> (x+y=w2411:u64)
                n467 = Compound Arithmetic op=ADD("BD 1 Frequency 1", w2397, w2409) -> (w2412:u64)
                "BD1 Frequency Out 1" <- w2412
              }
              frame #1 {
                # "Trap 2"
                n468 = case shown="True" "FB On/Off Set 2" {
                  tunnel: [w2549 w2550] -> w2545
                  tunnel: "BD 1 Amplitude 2" -> [w2549 _]
                  frame #0 {
                  }
                  frame #1 {
                    n469 = local read "AI2 Y Sum Set 2"() -> (w2555:i16)
                    n470 = call "Slower PID.vi"("process variable"=w2555, "reset?"="FB Reset Set 2", "setpoint"="FB Setpoint Set 2", "PID gains (x 2^8)"="FB Gains Set 2", "output range"="FB output range 2") -> ("output"=w2552:i16)  [unwired: 10 out]
                    n471 = To Unsigned Word Integer(number=w2552) -> (unsigned 16bit integer=w2550:u16)
                  }
                }
                "BD1 Frequency Out 2" <- "BD 1 Frequency 2"
              }
              frame #2 {
                # "Fluorescence period"
              }
            }
            n472 = feedback #47(w2288) -> (w2287:u32)
            n473 = Select(t=w2290, s="Interlace ON/OFF", f="Interlace Off Parameters") -> (s? t:f=w2328:u8)
            n474 = Subtract(x=w2288, y=w2287) -> (x-y=w2286:u32)
            n475 = Subtract "The error"(x=w2286, y=w2285) -> (x-y=w2263:u32)
            n476 = case shown="1, Default" w2328 {
              tunnel: ["DIO count 1 (ticks)" "DIO count 2 (ticks)" "DIO count 3 (ticks)"] -> w2284
              frame #0 {
              }
              frame #1 {
              }
              frame #2 {
              }
            }
            n477 = Number To Boolean Array(number=w2263) -> (Boolean array=w2264:bool[])
            n478 = Or Array Elements(Boolean array=w2264) -> (logical OR=w2262:bool)
            "DIO Late?" <- w2262
            n479 = Boolean To (0,1)(Boolean=w2262) -> (0, 1=w2269:i16)
            n480 = To Unsigned Word Integer(number=w2269) -> (unsigned 16bit integer=w2266:u16)
            n481 = feedback #48(u16 0) -> (w2267:u16)
            n482 = Add(x=w2266, y=w2267) -> (x+y=w2265:u16)
            "DIO Late Counter" <- w2265
            n483 = Subtract(x=w2284, y=w2263) -> (x-y=w2283:u32)
            n484 = Split Number(x=w2325) -> (hi(x)=w2324:u32, lo(x)=w2323:u32)
            n485 = Split Number(x=w2314) -> (hi(x)=w2319:u32, lo(x)=w2318:u32)
            n486 = Boolean To (0,1)(Boolean="+ phase (DIO)") -> (0, 1=w2280:i16)
            n487 = Split Number(x=w2324) -> (lo(x)=w2322:u16)  [unwired: 1 out]
            n488 = Split Number(x=w2323) -> (hi(x)=w2321:u16, lo(x)=w2320:u16)
            n489 = Split Number(x=w2319) -> (lo(x)=w2317:u16)  [unwired: 1 out]
            n490 = Split Number(x=w2318) -> (hi(x)=w2316:u16, lo(x)=w2315:u16)
            n491 = Split Number(x=w2273) -> (hi(x)=w2275:u8, lo(x)=w2274:u8)
            n492 = Split Number(x=w2270) -> (hi(x)=w2272:u8, lo(x)=w2271:u8)
            n493 = Split Number(x=w2322) -> (hi(x)=w2312:u8, lo(x)=w2311:u8)
            n494 = Split Number(x=w2321) -> (hi(x)=w2310:u8, lo(x)=w2309:u8)
            n495 = Split Number(x=w2317) -> (hi(x)=w2305:u8, lo(x)=w2304:u8)
            n496 = Split Number(x=w2320) -> (hi(x)=w2308:u8, lo(x)=w2307:u8)
            n497 = Split Number(x=w2316) -> (hi(x)=w2303:u8, lo(x)=w2302:u8)
            n498 = Split Number(x=w2315) -> (hi(x)=w2301:u8, lo(x)=w2300:u8)
            n499 = Multiply(x=w2280, y="Phase count adjustment (DIO)") -> (x*y=w2276:i16)
            n500 = feedback #49(i16 0) -> (w2278:i16)
            n501 = Subtract(x=w2278, y=w2276) -> (x-y=w2277:i16)
            "DIO Relative phase" <- w2277
            n502 = Add(x=w2283, y=w2276) -> (x+y=w2282:u32)
            n503 = Build Array "BD 1 A Stack"(w2275, w2274) -> (w2297:u8[])
            n504 = Build Array "BD 2 A Stack"(w2272, w2271) -> (w2296:u8[])
            n505 = Build Array "BD 1 nu Stack"(w2312, w2311, w2310, w2309, w2308, w2307) -> (w2306:u8[])
            n506 = Build Array "BD 2 nu Stack"(w2305, w2304, w2303, w2302, w2301, w2300) -> (w2299:u8[])
            n507 = case shown="2" w2313 {
              tunnel: [w2389 w2392] -> w2295
              tunnel: [u8 10 u8 4] -> w2298
              tunnel: "Swap F1 and F2" -> [w2390 w2392]
              frame #0 {
                # "F2"
                n508 = Not(x=w2390) -> (.not. x?=w2389:bool)
              }
              frame #1 {
                # "low chooses F1"
                # "F1"
              }
            }
            n509 = case "If FPGA is controlling (toggling) RF synth" shown="True" w2294 {
              tunnel: w2306 -> [_ w2342]
              tunnel: w2299 -> [_ w2341]
              tunnel: w2298 -> [_ w2340]
              tunnel: w2297 -> [_ w2339]
              tunnel: w2296 -> [_ w2338]
              frame #0 {
              }
              frame #1 {
                # "Write next amp.\n(wait until beginning of next loop iteration to update)"
                n510 = flat-sequence "Update the next F1 and F2 frequency value (the actual frequency won't change until FSK is switched).\nThen load the next amplitude value into buffer, but don't update it until the next cycle." {
                  tunnel: w2342 -> [w2345]
                  tunnel: w2341 -> [w2344]
                  tunnel: w2340 -> [w2343]
                  tunnel: w2339 -> [w2382]
                  tunnel: w2338 -> [w2381]
                  frame #0 {
                    n511 = for {
                      tunnel: w2345 -> [w2351] mode=indexing
                      tunnel: w2344 -> [w2350] mode=indexing
                      tunnel: w2343 -> [w2348]
                      i -> [w2349]
                      # "Write next freq."
                      n512 = To Unsigned Byte Integer(number=w2349) -> (unsigned 8bit integer=w2346:u8)
                      n513 = Add(x=w2348, y=w2346) -> (x+y=w2347:u8)
                      n514 = call "write to RF synth bd.vi"("Address Byte"=w2347, "BD 2 Byte"=w2350, "BD 1 Byte"=w2351) -> ()
                    }
                  }
                  frame #1 {
                    # "send udclk high"
                    n515 = xnode "FPGA I/O Node"("Connector1/DIO30"=TRUE ("Connector1/DIO15")) -> ()  [unwired: 1 in, 1 out]
                  }
                  frame #2 {
                    n516 = xnode "FPGA I/O Node"("Connector1/DIO30"=FALSE ("Connector1/DIO15")) -> ()  [unwired: 1 in, 1 out]
                  }
                  frame #3 {
                    n517 = for {
                      tunnel: w2382 -> [w2388] mode=indexing
                      tunnel: w2381 -> [w2387] mode=indexing
                      tunnel: u8 33 -> [w2385]
                      i -> [w2386]
                      n518 = To Unsigned Byte Integer(number=w2386) -> (unsigned 8bit integer=w2383:u8)
                      n519 = Add(x=w2385, y=w2383) -> (x+y=w2384:u8)
                      n520 = call "write to RF synth bd.vi"("Address Byte"=w2384, "BD 2 Byte"=w2387, "BD 1 Byte"=w2388) -> ()
                    }
                  }
                }
              }
            }
          }
        }
      }
    }
  }
  n521 = node-c288(w4) -> ()
